vi "GetNodeRef.vi"(8 "error in (no error)":errorcluster, 10 "Node Name":string, 11 "DirectedGraphWorldMap in":refnum<class "NI_Robotics_DirectedGraphWorldMap.lvclass">) -> (0 "error out":errorcluster, 1 "found":bool, 2 "Node ref":refnum<data-value>, 3 "DirectedGraphWorldMap out":refnum<class "NI_Robotics_DirectedGraphWorldMap.lvclass">)   [LabVIEW 2017, in "NI_Robotics_DirectedGraphWorldMap.lvclass"]
uses:
  <vilib>/robotics/Navigation/shared/WorldMap/DirectedGraphWorldMap/NI_Robotics_DirectedGraphWorldMap.lvclass
  <vilib>/robotics/Navigation/shared/MapNode/DirectedGraphMapNode/NI_Robotics_DirectedGraphMapNode.lvclass
  <vilib>/robotics/Navigation/shared/WorldMap/DirectedGraphWorldMap/NI_Robotics_DirectedGraphWorldMap.lvclass/NI_Robotics_DirectedGraphWorldMap.ctl
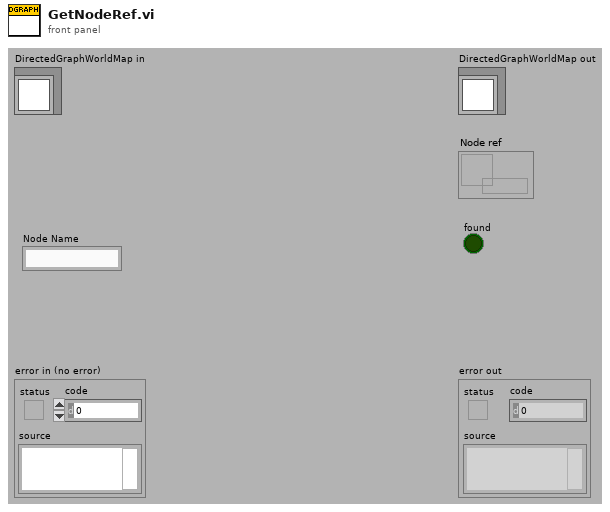
[diagram p1: front panel]
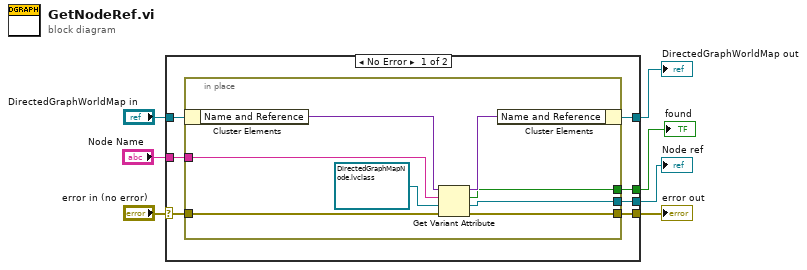
[diagram p0: block diagram]
diagram:
  n1 = case shown="No Error" "error in (no error)" {
    selector: "error in (no error)" -> [w11 w24]
    tunnel: [w10 w24] -> w6
    tunnel: [w13 w23] -> w4
    tunnel: "DirectedGraphWorldMap in" -> [w14 w23]
    tunnel: "Node Name" -> [w12 _]
    tunnel: [w9 _] -> w2
    tunnel: [w8 _] -> w1
    frame No Error {
      n2 = in-place {
        in-place-border: w12 -> [w20]
        in-place-border: [w19] -> w8
        in-place-border: [w17] -> w9
        in-place-border: w11 -> [w16]
        in-place-border: [w15] -> w10
        n3 = in-place-cluster #1(w14) -> ("Name and Reference"=w22:variant)
        n4 = Get Variant Attribute(Variant=w22, name=w20, default value (empty Variant)=refnum<data-value> refnum ("Node ref"), error in=w16) -> (duplicate Variant=w21:variant, found=w19:bool, value=w17:refnum<data-value>, error out=w15:errorcluster)
        n5 = in-place-cluster #1("Name and Reference"=w21) -> (w13:refnum<class "NI_Robotics_DirectedGraphWorldMap.lvclass">)
      }
    }
    frame Error {
    }
  }
  "error out" <- w6
  "DirectedGraphWorldMap out" <- w4
  "Node ref" <- w2
  "found" <- w1
